vi "MQTT_Simple_Connect_and_Subscribe.vi"() -> ()   [LabVIEW 2019, in "MQTT_Functions.lvlib"]
doc: "A basic client example that connects to a server, subscribes to a variety of topics and receives responses for the topics. \n\n© 2015 - daq.io, LLC - Peter Adelhardt"
uses:
  MQTT_Functions.lvlib
  Controls/QoS.ctl
  Controls/Retain_Flag.ctl
  Controls/DUP_Flag.ctl
  Controls/MessageType.ctl
  Controls/Connect_Flags.ctl
  Controls/Connection_Return_Codes.ctl
  Controls/MQTT_Broker_Details.ctl
panel:
  in  "MQTT Broker Details":T1={"address (IP)"="test.mosquitto.org", "port"=1883}
  out "Messages":T3(array[cluster])
  in  "Stop Reading":bool
  in  "Subscription Info Array":cluster{"Topic":string, "QoS":T4}[](array[cluster])=[{"Topic"="testtopic/LVMQTT", "QoS"=enum."At most once"}]
  out "Granted QoS Levels":T4[](array[typedef])
  out "Connection Status":T5=enum."Connection refused: Server unavailable"
  in  "Connect Flags":T6
  in  "Client ID":string="LVSubscribeClient"
  out "error out":errorcluster
  in  "error in (no error)":errorcluster
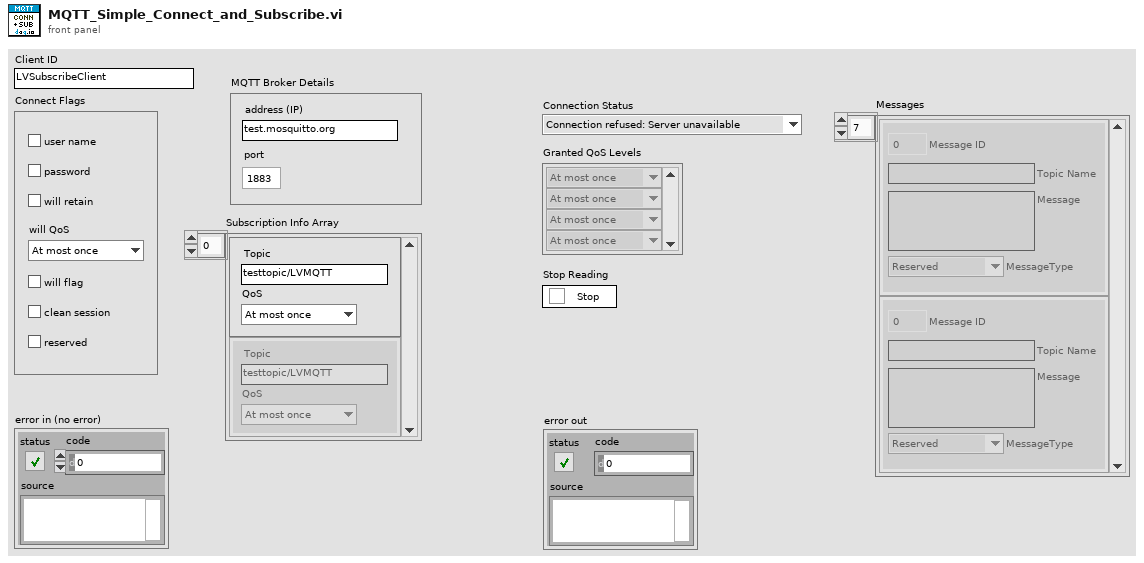
[diagram p1: front panel]
types:
  T1 = typedef "MQTT_Functions.lvlib/MQTT_Broker_Details.ctl" = cluster{"address (IP)":string, "port":u16}
  T2 = typedef "MQTT_Functions.lvlib/MessageType.ctl" = enum32{"Reserved", "CONNECT", "CONNACK", "PUBLISH", "PUBACK", "PUBREC", "PUBREL", "PUBCOMP", "SUBSCRIBE", "SUBACK", "UNSUBSCRIBE", "UNSUBACK", "PINGREQ", "PINGRESP", "DISCONNECT", "Reserved2"}
  T3 = cluster{"Message ID":u16, "Topic Name":string, "Message ":string, "MessageType":T2}[]
  T4 = typedef "MQTT_Functions.lvlib/QoS.ctl" = enum8{"At most once", "At least once", "Exactly once", "Reserved"}
  T5 = typedef "MQTT_Functions.lvlib/Connection_Return_Codes.ctl" = enum16{"Connection accepted", "Connection refused: unacceptable protocol version", "Connection refused: identifier rejected", "Connection refused: Server unavailable", "Connection refused: bad user name or password", "Connection refused: not authorized"}
  T6 = typedef "MQTT_Functions.lvlib/Connect_Flags.ctl" = cluster{"user name":bool, "password":bool, "will retain":bool, "will flag":bool, "clean session":bool, "reserved":bool, "will QoS":T4}
  T7 = cluster{"Message ID":u16, "Topic Name":string, "Message":string, "MessageType":T2}[]
  T8 = typedef "MQTT_Functions.lvlib/DUP_Flag.ctl" = bool
  T9 = typedef "MQTT_Functions.lvlib/Retain_Flag.ctl" = bool
  T10 = cluster{"QoS":T4, "DUP":T8, "Retain":T9, "Keep Alive (sec)":u16}
  T11 = cluster{"Message ID":u16, "Topic Name":string, "Message":string, "MessageType":T2}
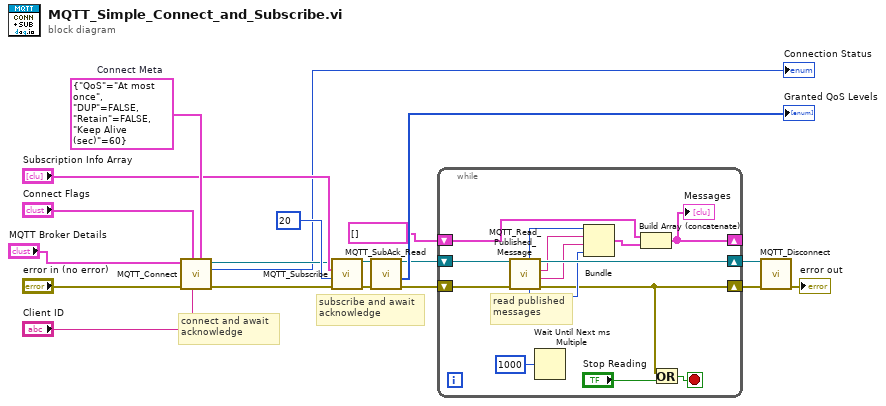
[diagram p0: block diagram]
diagram:
  w16 = T10 {"QoS"=enum."At most once", "DUP"=FALSE, "Retain"=FALSE, "Keep Alive (sec)"=60}  # Connect Meta
  # "connect and await\nacknowledge"
  # "subscribe and await\nacknowledge"
  n1 = call "MQTT_Connect.vi"("Connect Meta"=w16, "Client ID"="Client ID", "Connect Flags"="Connect Flags", "error in (no error)"="error in (no error)", "MQTT Broker Details"="MQTT Broker Details") -> ("error out"=w2:errorcluster, "Connection Status"=→"Connection Status":T5, "connection ID out"=w4:refnum<k5>)  [unwired: 4 in]
  n2 = call "MQTT_Subscribe.vi"("error in (no error)"=w2, "Message ID"=u16 20, "Subscription Info Array"="Subscription Info Array", "connection ID"=w4) -> ("error out"=w12:errorcluster, "connection ID out"=w13:refnum<k5>)  [unwired: 6 in]
  n3 = call "MQTT_SubAck_Read.vi"("error in (no error)"=w12, "connection ID"=w13) -> ("error out"=w10:errorcluster, "Granted QoS Levels"=→"Granted QoS Levels":T4[], "connection ID out"=w9:refnum<k5>)  [unwired: 7 in]
  n4 = while {
    shift-right: [w20] -> _
    shift-left: T7 [] ("Array") -> [w22]
    shift-right: [w23] -> w7
    shift-left: w10 -> [w33]
    shift-right: [w31] -> w8
    shift-left: w9 -> [w32]
    stop <- w25 stop-if-true
    # "read published\nmessages"
    n5 = call "MQTT_Read_Published_Message.vi"("error in (no error)"=w33, "connection ID"=w32) -> ("error out"=w23:errorcluster, "Message"=w28:string, "Topic Name"=w29:string, "connection ID out"=w31:refnum<k5>, "MessageType"=w27:T2, "Message ID"=w30:u16)  [unwired: 4 in]
    n6 = Wait Until Next ms Multiple(millisecond multiple=u32 1000) -> ()  [unwired: 1 out]
    n7 = Bundle("Message ID"=w30, "Topic Name"=w29, "Message"=w28, "MessageType"=w27) -> (w21:T11)  [unwired: 1 in]
    n8 = Build Array (concatenate)(w22, w21) -> (w20:T7)
    "Messages" <- w20
    n9 = Or(x=w23, y="Stop Reading") -> (x .or. y?=w25:bool)
  }
  n10 = call "MQTT_Disconnect.vi"("error in (no error)"=w7, "connection ID"=w8) -> ("error out"=→"error out":errorcluster)  [unwired: 9 in]
